vi "PCF8591_Initial.vi"(8 "error in (no error)":errorcluster) -> (0 "error out":errorcluster)   [LabVIEW 2014, in "QwaveSys Raspberry Pi Library.lvlib"]
uses:
  QwaveSys Raspberry Pi Library.lvlib
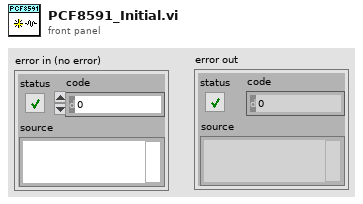
[diagram p1: front panel]
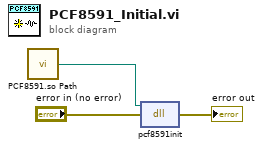
[diagram p0: block diagram]
diagram:
  n1 = call "PCF8591.so Path.vi"() -> ("PCF8591.so Path"=w1:path)  [unwired: 5 in]
  n2 = dll-call lib="pcf8591.so" fn="pcf8591init"(path in=w1, error in="error in (no error)") -> (error out=→"error out":errorcluster)  [unwired: 2 in, 1 out]
